vi "GSP_Manager_F2.vi"() -> ()   [LabVIEW 2015]
uses:
  SystemUtil/Command.ctl
  SystemUtil/ScriptArray.ctl
  SystemUtil/Script.ctl
  SystemUtil/MotorStates.ctl
  SystemUtil/ThreadStates.ctl
  Log/LogItem.ctl
  GSP_F2_Global.vi
  GUI/GSP_GUI_global.vi
panel:
  in  "Secondary Filter":i32(ring) items=["<NO FILTER>", "GG495new", "S8612", "U", "GG455", "GG385"]
  out "Last Error":errorcluster
  in  "CommandQ":string
  # "Secondary Filter"
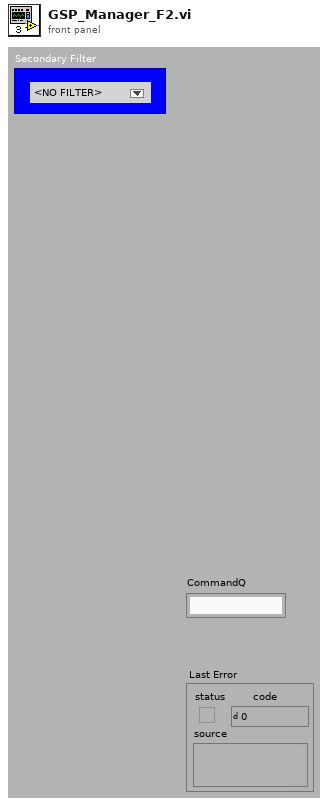
[diagram p1: front panel]
types:
  T1 = typedef "Command.ctl" = cluster{"Command":string, "Parameter":string}
  T2 = typedef "ScriptArray.ctl" = T3[]
  T3 = typedef "Script.ctl" = cluster{"Current Step":i32, "Commands":cluster{"Command":string, "Parameters":string}[]}
  T4 = cluster{"Move Mem Address":i32, "Home Mem Address":i32}
  T5 = typedef "MotorStates.ctl" = enum16{"Ready", "Moving", "Uninitialized", "Error"}
  T6 = typedef "ThreadStates.ctl" = enum16{"Waiting", "Scripting", "Uninitialized", "Error"}
  T7 = typedef "LogItem.ctl" = cluster{"error in (no error)":errorcluster, "Source":string, "Comment ":string}
  T8 = enum16{"Launch", "Log", "Open", "Close", "Shutdown"}
  T9 = enum16{"POL (0)", "CPL (1)", "HLT (2)", "STP (3)", "RST (4)", "RVN (5)", "RPB (6)", "CLP (8)", "SDL (9)", "RUN (10)", "WRI (11)", "RRG (12)", "SPR (13)", "LPR (14)", "VMI (15)", "SSP (17)", "SSE (18)", "RIS (20)", "RIO (21)", "IMW (25)", "END (128)", "MAV (134)", "MRV (135)", "JRE (137)", "WCL (138)", "WCW (139)", "DLY (140)", "WDL (141)", "GCL (142)", "GOP (143)", "ZTG (144)", "ZTP (145)", "TTP (146)", "CME (147)", "CTC (148)", "TQL (149)", "AHC (150)", "ERL (151)", "OLP (152)", "WRP (154)", "IDT (155)", "LRP (156)", "VMP (159)", "RAV (160)", "RRV (161)", "JMP (162)", "JOI (162)", "CIS (163)", "CKS (164)", "CLC (165)", "KMC (167)", "MCT (168)", "FLC (169)", "EEM (170)", "DDB (171)", "DEM (171)", "PAC (172)", "ADL (173)", "BRT (174)", "MAT (176)", "MRT (177)", "RAT (178)", "RRT (179)", "SSD (180)", "KMR (181)", "KED (182)", "KDD (183)", "DIR (184)", "PRO (185)", "SIF (186)", "EDL (187)", "CIO (188)", "MDS (189)", "MDC (190)", "MDT (191)", "SEE (192)", "ARI (193)", "WBS (194)", "SCF (195)", "RSM (196)", "RLM (197)", "RSN (198)", "RLN (199)", "PCL (201)", "PCI (201)", "PRT (202)", "PRI (202)", "WBE (204)", "SOB (205)", "COB (206)", "ACR (207)", "PLR (208)", "CAI (211)", "LVT (212)", "OVT (213)", "MTT (214)", "CLC (215)", "PIM (216)", "VIM (217)", "TIM (218)", "AHM (219)", "SSL (221)", "TRU (222)", "RSD (223)", "EMT (225)", "DMT (226)", "EMD (227)", "DMD (228)", "HSM (229)", "AHD (230)", "PCM (231)", "PCG (232)", "XRV (233)", "XAV (234)", "XRT (235)", "XAT (236)", "GOC (237)", "JNA (238)", "JOR (239)", "PMC (240)", "PMV (241)", "PMX (242)", "DLC (243)", "SLC (244)", "PCP (245)", "ATR (248)", "PMO (249)", "JAN (250)", "EDH (251)", "DIF (252)", "IMS (253)", "IMQ (254)"}
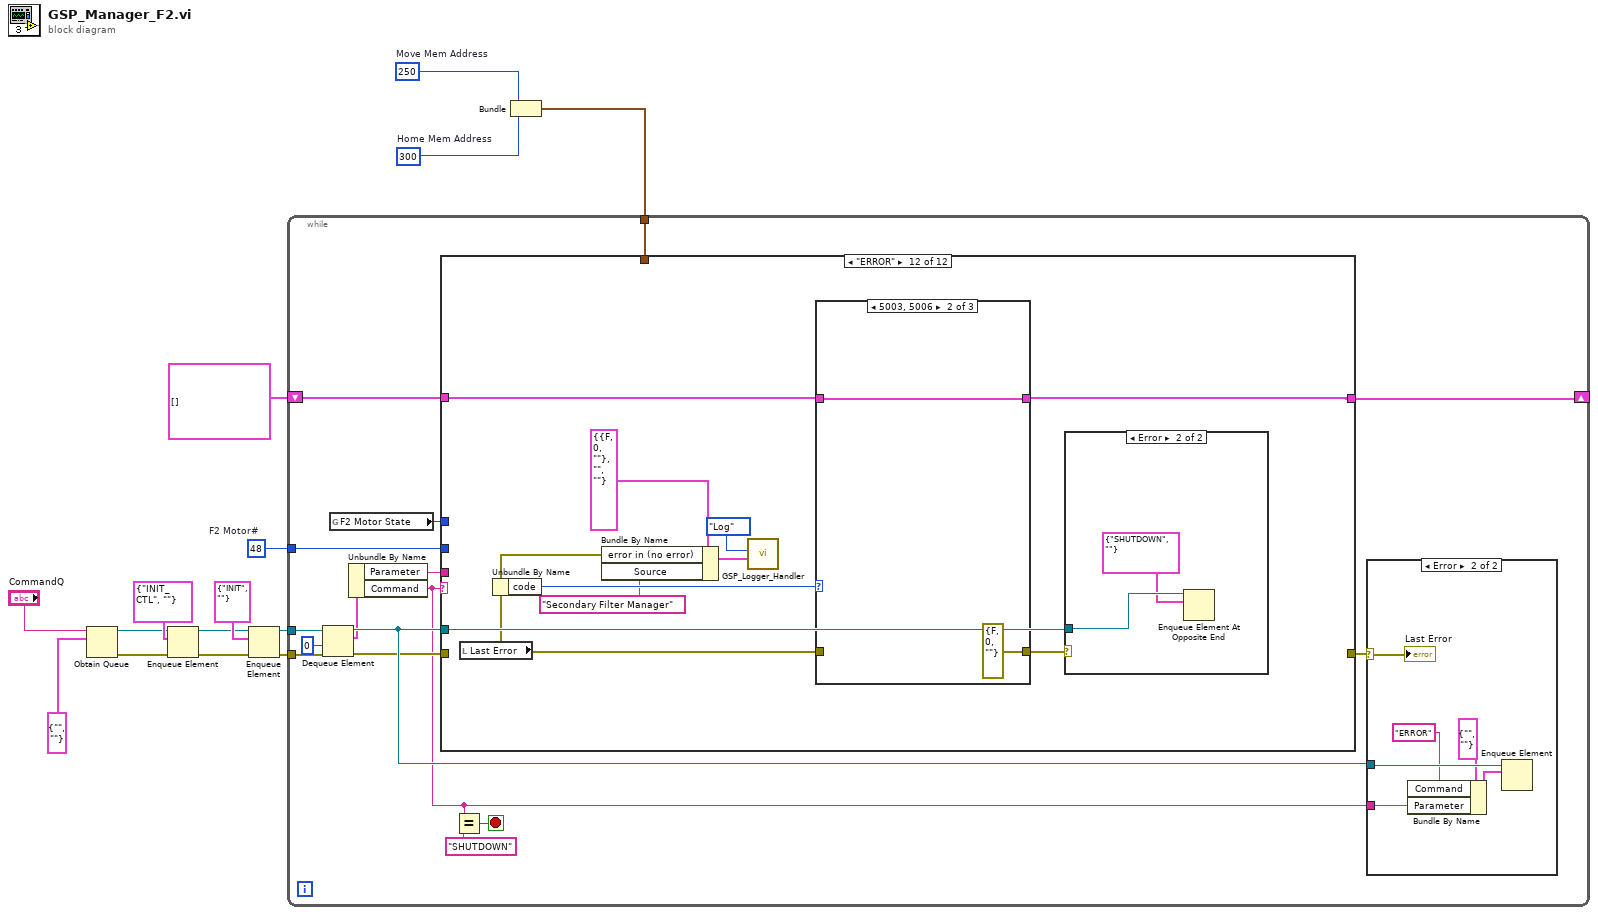
[diagram p0: block diagram]
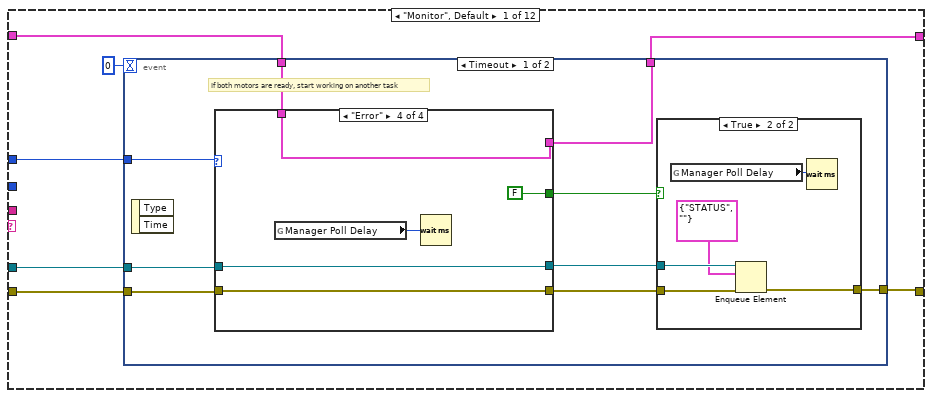
[diagram p3: hidden frame]
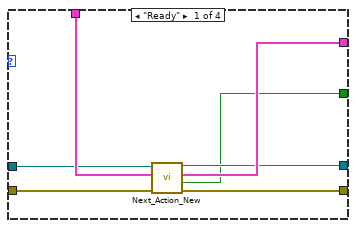
[diagram p5: hidden frame]
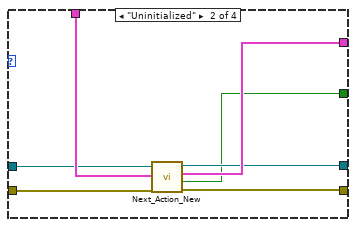
[diagram p6: hidden frame]
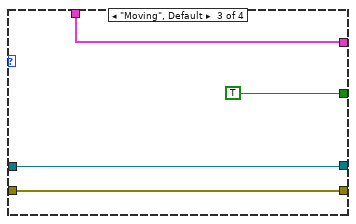
[diagram p7: hidden frame]
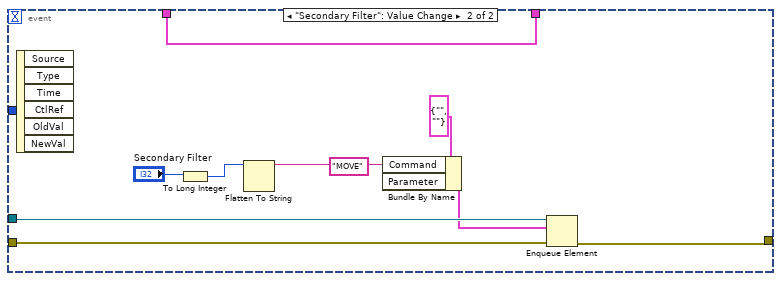
[diagram p8: hidden frame]
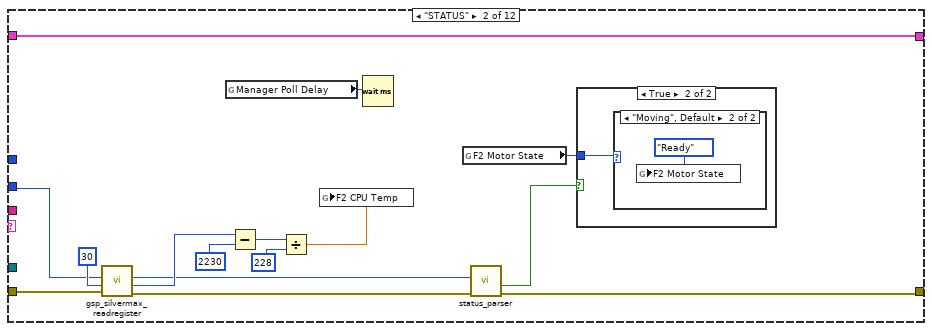
[diagram p9: hidden frame]
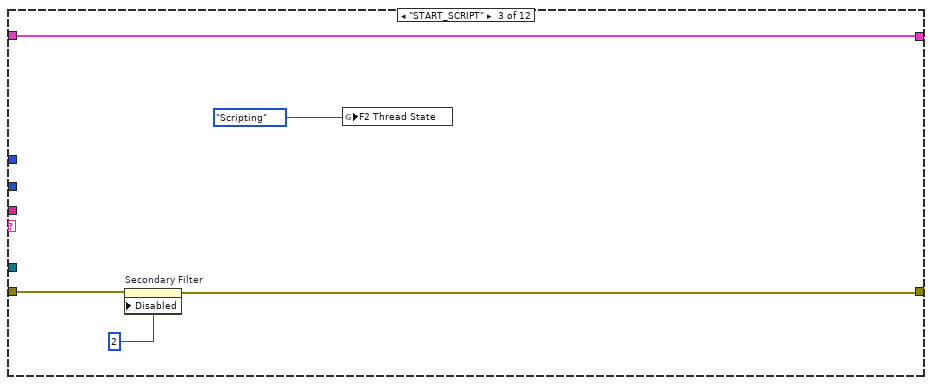
[diagram p12: hidden frame]
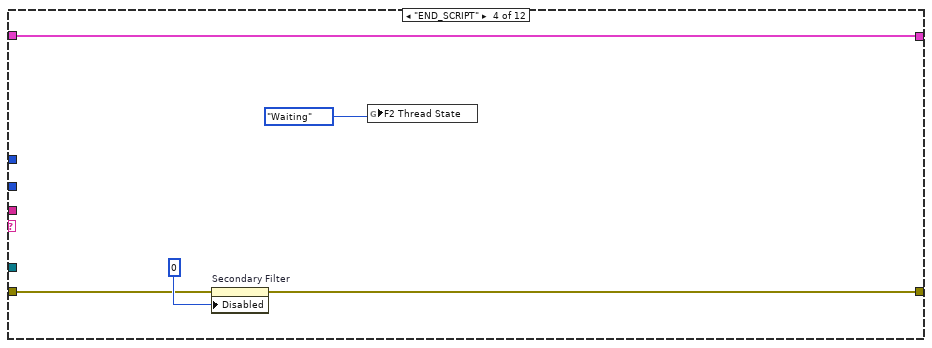
[diagram p13: hidden frame]
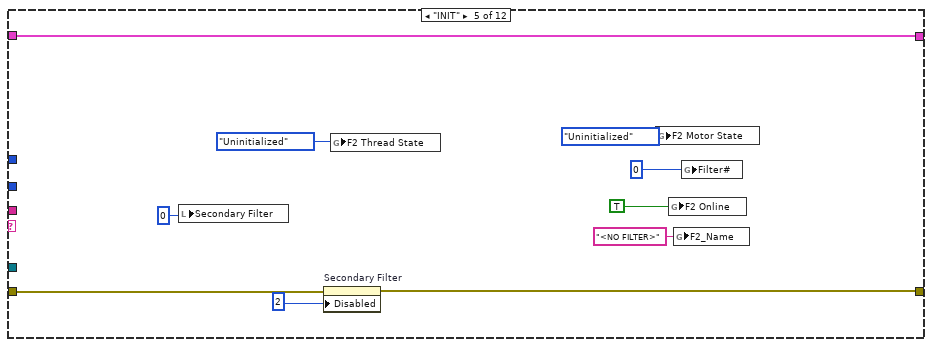
[diagram p14: hidden frame]
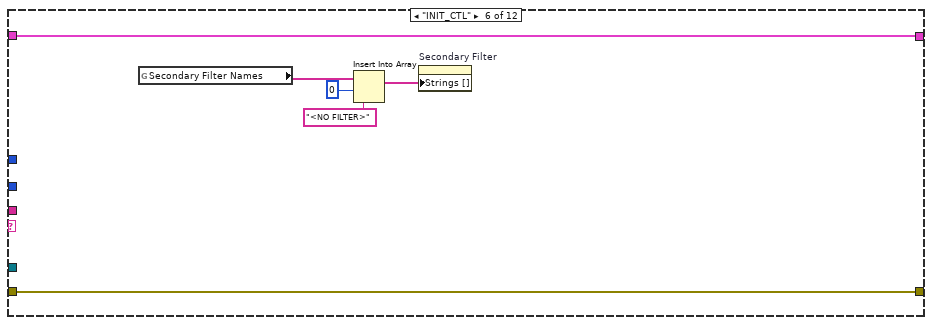
[diagram p15: hidden frame]
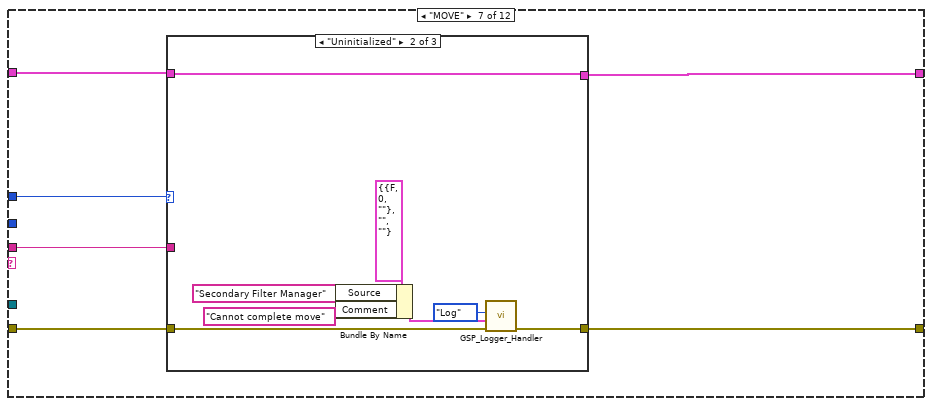
[diagram p16: hidden frame]
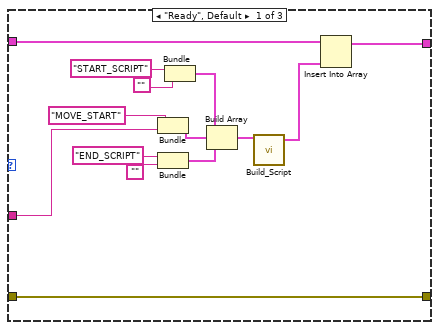
[diagram p17: hidden frame]
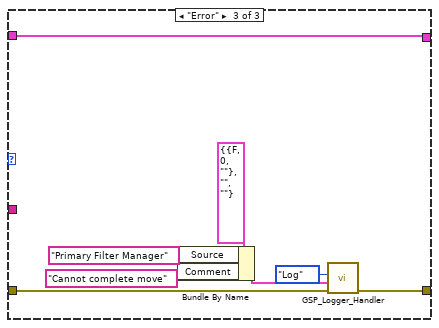
[diagram p18: hidden frame]
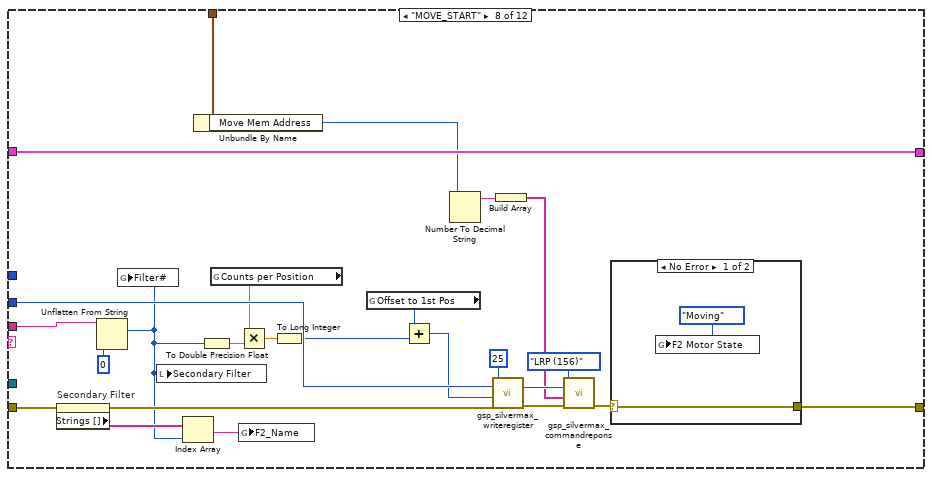
[diagram p19: hidden frame]
diagram:
  w7 = 300  # Home Mem Address
  w8 = 250  # Move Mem Address
  w12 = u8 48  # F2 Motor#
  n1 = Obtain Queue(name (unnamed)="CommandQ", element data type=T1 {"Command"="", "Parameter"=""} ("Command")) -> (queue out=w2:refnum<queue>, error out=w1:errorcluster)  [unwired: 3 in, 1 out]
  n2 = Enqueue Element(queue=w2, element=T1 {"Command"="INIT_CTL", "Parameter"=""}, error in (no error)=w1) -> (queue out=w4:refnum<queue>, error out=w3:errorcluster)  [unwired: 1 in, 1 out]
  n3 = Enqueue Element(queue=w4, element=T1 {"Command"="INIT", "Parameter"=""}, error in (no error)=w3) -> (queue out=w15:refnum<queue>, error out=w14:errorcluster)  [unwired: 1 in, 1 out]
  n4 = Bundle("Move Mem Address"=w8, "Home Mem Address"=w7) -> (w6:T4)  [unwired: 1 in]
  n5 = while {
    tunnel: w15 -> [w31]
    tunnel: w14 -> [w30]
    tunnel: w12 -> [w25]
    shift-right: [w23] -> _
    shift-left: T2 [] ("Operations") -> [w24]
    tunnel: w6 -> [w16]
    stop <- w19 stop-if-true
    n6 = Dequeue Element(queue=w31, timeout in ms (-1)=0, error in (no error)=w30) -> (queue out=w28:refnum<queue>, element=w21:T1, error out=w26:errorcluster)  [unwired: 1 out]
    n7 = global read "GSP_F2_Global.vi" "F2 Motor State"() -> (w17:T5)
    n8 = Unbundle By Name(w21) -> ("Parameter"=w20:string, "Command"=w18:string)
    n9 = case shown="\"ERROR\"" w18 {
      tunnel: w26 -> [w43 w97 w113 w117 w125 w131 w139 w176 w205 w221 w223 _]
      tunnel: w28 -> [w44 _ _ _ _ _ _ _ w204 _ _ w245]
      tunnel: [w39 w106 w111 w116 w123 w131 w138 w188 w200 w221 w230 _] -> w29
      tunnel: w25 -> [_ w95 _ _ _ _ _ w191 _ _ w232 _]
      tunnel: w24 -> [w42 w105 w114 w119 w128 w130 w141 w184 w206 w220 w227 w238]
      tunnel: [w41 w105 w114 w119 w128 w130 w140 w184 w206 w219 w227 w237] -> w23
      tunnel: w20 -> [_ _ _ _ _ _ w137 w183 _ _ _ _]
      tunnel: w17 -> [w40 _ _ _ _ _ w136 _ _ _ _ _]
      tunnel: w16 -> [_ _ _ _ _ _ _ w178 _ _ w226 _]
      frame "Monitor", Default {
        n10 = event shown="[0] Timeout" {
          selector: _ -> [_ _]
          dyn-events: _ -> [_ _]
          timeout: 0 -> [_ _]
          tunnel: w44 -> [w53 w88]
          tunnel: w43 -> [w52 w89]
          tunnel: w42 -> [w51 w92]
          tunnel: [w50 w92] -> w41
          tunnel: w40 -> [w49 _]
          tunnel: [w45 w83] -> w39
          event Timeout {
            # "If both motors are ready, start working on another task"
            n11 = event-data() -> ()  [unwired: 1 in, 2 out]
            n12 = case shown="\"Error\"" w49 {
              tunnel: w53 -> [w62 w69 w76 w79]
              tunnel: w52 -> [w66 w73 w75 w81]
              tunnel: [w63 w70 w75 w81] -> w48
              tunnel: w51 -> [w65 w72 w77 w82]
              tunnel: [w64 w71 w77 w82] -> w50
              tunnel: [w61 w68 w76 w79] -> w47
              tunnel: [w60 w67 TRUE FALSE] -> w46
              frame "Ready" {
                n13 = call "Next_Action_New.vi"("error in (no error)"=w66, "Operations"=w65, "queue in"=w62) -> ("error out"=w63:errorcluster, "No command?"=w60:bool, "Operations Out"=w64:T2, "queue out"=w61:refnum<queue>)  [unwired: 1 in]
              }
              frame "Uninitialized" {
                n14 = call "Next_Action_New.vi"("error in (no error)"=w73, "Operations"=w72, "queue in"=w69) -> ("error out"=w70:errorcluster, "No command?"=w67:bool, "Operations Out"=w71:T2, "queue out"=w68:refnum<queue>)  [unwired: 1 in]
              }
              frame "Moving", Default {
              }
              frame "Error" {
                n15 = global read "GSP_GUI_global.vi" "Manager Poll Delay"() -> (w80:u32)
                n16 = Wait (ms)(milliseconds to wait=w80) -> ()  [unwired: 1 out]
              }
            }
            n17 = case shown="True" w46 {
              tunnel: w48 -> [w54 w59]
              tunnel: w47 -> [_ w58]
              tunnel: [w54 w57] -> w45
              frame False {
              }
              frame True {
                n18 = global read "GSP_GUI_global.vi" "Manager Poll Delay"() -> (w56:u32)
                n19 = Enqueue Element(queue=w58, element=T1 {"Command"="STATUS", "Parameter"=""}, error in (no error)=w59) -> (error out=w57:errorcluster)  [unwired: 1 in, 2 out]
                n20 = Wait (ms)(milliseconds to wait=w56) -> ()  [unwired: 1 out]
              }
            }
          }
          event "Secondary Filter": Value Change {
            n21 = event-data() -> ()  [unwired: 1 in, 6 out]
            n22 = To Long Integer(number="Secondary Filter") -> (32bit integer=w84:i32)
            n23 = Flatten To String(anything=w84) -> (data string=w90:string)  [unwired: 3 in, 2 out]
            n24 = Bundle By Name(cluster=T1 {"Command"="", "Parameter"=""} ("element"), "Command"="MOVE" ("element"), "Parameter"=w90) -> (w86:T1)
            n25 = Enqueue Element(queue=w88, element=w86, error in (no error)=w89) -> (error out=w83:errorcluster)  [unwired: 1 in, 2 out]
          }
        }
      }
      frame "STATUS" {
        n26 = call "gsp_silvermax_readregister.vi"("error in (no error)"=w97, "Register# (0)"=u8 30, "Motor #"=w95) -> ("error out"=w96:errorcluster, "Register Value"=w102:i32, "Motor # dup"=w94:u8)  [unwired: 2 in, 2 out]
        n27 = global read "GSP_GUI_global.vi" "Manager Poll Delay"() -> (w104:u32)
        n28 = Subtract(x=w102, y=2230) -> (x-y=w101:i32)
        n29 = Divide(x=w101, y=228) -> (x/y=w98:dbl)
        n30 = global write "GSP_F2_Global.vi" "F2 CPU Temp"(w98) -> ()
        n31 = Wait (ms)(milliseconds to wait=w104) -> ()  [unwired: 1 out]
        n32 = global read "GSP_F2_Global.vi" "F2 Motor State"() -> (w93:T5)
        n33 = call "status_parser.vi"("error in (no error)"=w96, "Motor #"=w94) -> ("error out"=w106:errorcluster, "Program Complete?"=w107:bool)  [unwired: 3 in, 1 out]
        n34 = case shown="True" w107 {
          tunnel: w93 -> [_ w108]
          frame False {
          }
          frame True {
            n35 = case shown="\"Moving\", Default" w108 {
              frame "Uninitialized" {
              }
              frame "Moving", Default {
                n36 = global write "GSP_F2_Global.vi" "F2 Motor State"(MotorStates."Ready" ("Mode")) -> ()
              }
            }
          }
        }
      }
      frame "START_SCRIPT" {
        n37 = property on="Secondary Filter" class="Ring (strict)"(error in=w113, "Disabled"=u8 2) -> (error out=w111:errorcluster)  [unwired: 1 in, 1 out]
        n38 = global write "GSP_F2_Global.vi" "F2 Thread State"(ThreadStates."Scripting" ("Thread state")) -> ()
      }
      frame "END_SCRIPT" {
        n39 = property on="Secondary Filter" class="Ring (strict)"(error in=w117, "Disabled"=u8 0) -> (error out=w116:errorcluster)  [unwired: 1 in, 1 out]
        n40 = global write "GSP_F2_Global.vi" "F2 Thread State"(ThreadStates."Waiting" ("Thread state")) -> ()
      }
      frame "INIT" {
        n41 = local write "Secondary Filter"(0 ("Value")) -> ()
        n42 = property on="Secondary Filter" class="Ring (strict)"(error in=w125, "Disabled"=u8 2) -> (error out=w123:errorcluster)  [unwired: 1 in, 1 out]
        n43 = global write "GSP_F2_Global.vi" "F2 Thread State"(ThreadStates."Uninitialized" ("Thread state")) -> ()
        n44 = global write "GSP_F2_Global.vi" "F2 Motor State"(MotorStates."Uninitialized" ("Mode")) -> ()
        n45 = global write "GSP_F2_Global.vi" "F2 Online"(TRUE ("CS Online")) -> ()
        n46 = global write "GSP_F2_Global.vi" "F2_Name"("<NO FILTER>" ("F2_Name")) -> ()
        n47 = global write "GSP_F2_Global.vi" "Filter#"(0 ("Filter Position")) -> ()
      }
      frame "INIT_CTL" {
        n48 = global read "GSP_GUI_global.vi" "Secondary Filter Names"() -> (w133:string[])
        n49 = Insert Into Array(array=w133, index=0, new element="<NO FILTER>" ("new element/subarray")) -> (w132:string[])
        n50 = property on="Secondary Filter" class="Ring (strict)"("Strings []"=w132) -> ()  [unwired: 2 in, 2 out]
      }
      frame "MOVE" {
        n51 = case shown="\"Uninitialized\"" w136 {
          tunnel: w141 -> [w155 w163 w171]
          tunnel: [w154 w163 w171] -> w140
          tunnel: w139 -> [w153 w162 w170]
          tunnel: [w153 w161 w169] -> w138
          tunnel: w137 -> [w147 _ _]
          frame "Ready", Default {
            n52 = Bundle("MOVE_START", "Parameter"=w147) -> (w146:cluster{string, "Parameter":string})  [unwired: 1 in]
            n53 = Bundle("END_SCRIPT", "") -> (w149:cluster{string, string})  [unwired: 1 in]
            n54 = Bundle("START_SCRIPT", "") -> (w142:cluster{string, string})  [unwired: 1 in]
            n55 = Build Array(w142, w146, w149) -> (w148:cluster{string, "Parameter":string}[])
            n56 = call "Build_Script.vi"("Commands"=w148) -> ("script out"=w145:T3)  [unwired: 4 in]
            n57 = Insert Into Array(array=w155, new element=w145) -> (w154:T2)  [unwired: 1 in]
          }
          frame "Uninitialized" {
            n58 = Bundle By Name(cluster=T7 {"error in (no error)"={"status"=FALSE, "code"=0, "source"=""}, "Source"="", "Comment "=""} ("Log"), "Source"="Secondary Filter Manager", "Comment"="Cannot complete move") -> (w158:T7)
            n59 = call "GSP_Logger_Handler.vi"("error in (no error)"=w162, "Log"=w158, "Actions"=T8."Log") -> ("error out"=w161:errorcluster)  [unwired: 4 in]
          }
          frame "Error" {
            n60 = Bundle By Name(cluster=T7 {"error in (no error)"={"status"=FALSE, "code"=0, "source"=""}, "Source"="", "Comment "=""} ("Log"), "Source"="Primary Filter Manager", "Comment"="Cannot complete move") -> (w166:T7)
            n61 = call "GSP_Logger_Handler.vi"("error in (no error)"=w170, "Log"=w166, "Actions"=T8."Log") -> ("error out"=w169:errorcluster)  [unwired: 4 in]
          }
        }
      }
      frame "MOVE_START" {
        n62 = property on="Secondary Filter" class="Ring (strict)"(error in=w176) -> (error out=w174:errorcluster, "Strings []"=w175:string[])  [unwired: 1 in, 1 out]
        n63 = Unflatten From String(type=0, binary string=w183) -> (value=w173:i32)  [unwired: 3 in, 2 out]
        n64 = global write "GSP_F2_Global.vi" "Filter#"(w173) -> ()
        n65 = local write "Secondary Filter"(w173) -> ()
        n66 = Index Array(array=w175, index=w173) -> (element=w172:string)
        n67 = Unbundle By Name(w178) -> ("Move Mem Address"=w177:i32)
        n68 = To Double Precision Float(number=w173) -> (double precision float=w196:dbl)
        n69 = global read "GSP_F2_Global.vi" "Counts per Position"() -> (w187:dbl)
        n70 = Multiply(x=w187, y=w196) -> (x*y=w195:dbl)
        n71 = global write "GSP_F2_Global.vi" "F2_Name"(w172) -> ()
        n72 = To Long Integer(number=w195) -> (32bit integer=w181:i32)
        n73 = global read "GSP_F2_Global.vi" "Offset to 1st Pos"() -> (w179:i32)
        n74 = Add(x=w179, y=w181) -> (x+y=w180:i32)
        n75 = Number To Decimal String(number=w177) -> (decimal integer string=w186:string)  [unwired: 1 in]
        n76 = call "gsp_silvermax_writeregister.vi"("error in (no error)"=w174, "Register Value"=w180, "Motor #"=w191, "Register# (0)"=u8 25) -> ("error out"=w193:errorcluster, "Motor # dup"=w192:u8)  [unwired: 2 in]
        n77 = Build Array(w186) -> (w185:string[])
        n78 = call "gsp_silvermax_commandreponse.vi"("error in (no error)"=w193, "Parameters (none)"=w185, "Motor #"=w192, "Command"=T9."LRP (156)") -> ("error out"=w189:errorcluster)  [unwired: 3 out]
        n79 = case shown="No Error" w189 {
          selector: w189 -> [w198 w199]
          tunnel: [w198 w199] -> w188
          frame No Error {
            n80 = global write "GSP_F2_Global.vi" "F2 Motor State"(MotorStates."Moving" ("Mode")) -> ()
          }
          frame Error {
          }
        }
      }
      frame "SHUTDOWN" {
        n81 = Release Queue(queue=w204, error in (no error)=w205) -> (error out=w201:errorcluster)  [unwired: 1 in, 2 out]
        n82 = global write "GSP_F2_Global.vi" "F2 Thread State"(ThreadStates."Uninitialized" ("Thread state")) -> ()
        n83 = property on="Secondary Filter" class="Ring (strict)"(error in=w201, "Disabled"=u8 2) -> (error out=w200:errorcluster)  [unwired: 1 in, 1 out]
        n84 = stacked-sequence {
          tunnel: w200 -> [_]
          frame #0 {
            n85 = global write "GSP_F2_Global.vi" "F2 Online"(FALSE ("CS Online")) -> ()
          }
        }
      }
      frame "HOME" {
        n86 = Bundle("START_SCRIPT", "") -> (w208:cluster{string, string})  [unwired: 1 in]
        n87 = Bundle("HOME_START", "") -> (w214:cluster{string, string})  [unwired: 1 in]
        n88 = Bundle("END_SCRIPT", "") -> (w213:cluster{string, string})  [unwired: 1 in]
        n89 = Build Array(w208, w214, w213) -> (w212:cluster{string, string}[])
        n90 = call "Build_Script.vi"("Commands"=w212) -> ("script out"=w211:T3)  [unwired: 4 in]
        n91 = Insert Into Array(array=w220, new element=w211) -> (w219:T2)  [unwired: 1 in]
      }
      frame "HOME_START" {
        n92 = Unbundle By Name(w226) -> ("Home Mem Address"=w225:i32)
        n93 = local write "Secondary Filter"(0 ("Value")) -> ()
        n94 = global write "GSP_F2_Global.vi" "F2_Name"("<NO FILTER>" ("F2_Name")) -> ()
        n95 = Number To Decimal String(number=w225) -> (decimal integer string=w229:string)  [unwired: 1 in]
        n96 = Build Array(w229) -> (w228:string[])
        n97 = call "gsp_silvermax_commandreponse.vi"("error in (no error)"=w223, "Parameters (none)"=w228, "Motor #"=w232, "Command"=T9."LRP (156)") -> ("error out"=w233:errorcluster)  [unwired: 3 out]
        n98 = case shown="No Error" w233 {
          selector: w233 -> [w235 w236]
          tunnel: [w235 w236] -> w230
          frame No Error {
            n99 = global write "GSP_F2_Global.vi" "F2 Motor State"(MotorStates."Moving" ("Mode")) -> ()
          }
          frame Error {
          }
        }
      }
      frame "ERROR" {
        n100 = local read "Last Error"() -> (w240:errorcluster)
        n101 = Unbundle By Name(w240) -> ("code"=w246:i32)
        n102 = Bundle By Name(cluster=T7 {"error in (no error)"={"status"=FALSE, "code"=0, "source"=""}, "Source"="", "Comment "=""} ("Log"), "error in (no error)"=w240, "Source"="Secondary Filter Manager") -> (w242:T7)
        n103 = call "GSP_Logger_Handler.vi"("Log"=w242, "Actions"=T8."Log") -> ()  [unwired: 5 in, 1 out]
        n104 = case shown="5003, 5006" w246 {
          tunnel: w240 -> [_ _ _]
          tunnel: [errorcluster {"status"=FALSE, "code"=0, "source"=""} ("error IO") errorcluster {"status"=FALSE, "code"=0, "source"=""} ("error IO") errorcluster {"status"=FALSE, "code"=0, "source"=""} ("error IO")] -> w239
          tunnel: w238 -> [_ w255 w257]
          tunnel: [T2 [] ("Operations") w255 w257] -> w237
          frame 0, Default {
            n105 = global write "GSP_F2_Global.vi" "F2 Motor State"(MotorStates."Error" ("Mode")) -> ()
            n106 = property on="Secondary Filter" class="Ring (strict)"("Disabled"=u8 2) -> ()  [unwired: 2 in, 2 out]
            n107 = global write "GSP_F2_Global.vi" "F2 Thread State"(ThreadStates."Error" ("Thread state")) -> ()
          }
          frame 5003, 5006 {
          }
          frame 5013 {
          }
        }
        n108 = case shown="Error" w239 {
          tunnel: w245 -> [_ w248]
          frame No Error {
          }
          frame Error {
            n109 = Enqueue Element At Opposite End(queue=w248, element=T1 {"Command"="SHUTDOWN", "Parameter"=""}) -> ()  [unwired: 2 in, 3 out]
          }
        }
      }
    }
    n110 = Equal?(x=w18, y="SHUTDOWN") -> (x = y?=w19:bool)
    n111 = case shown="Error" w29 {
      selector: w29 -> [_ w36]
      tunnel: w28 -> [_ w37]
      tunnel: w18 -> [_ w33]
      frame No Error {
      }
      frame Error {
        n112 = Bundle By Name(cluster=T1 {"Command"="", "Parameter"=""} ("element"), "Command"="ERROR" ("element"), "Parameter"=w33) -> (w35:T1)
        n113 = Enqueue Element(queue=w37, element=w35) -> ()  [unwired: 2 in, 3 out]
        "Last Error" <- w36
      }
    }
  }
